vi "Do Core.vi"(8 "error in":errorcluster, 9 "Actor in":refnum<class "Actor.lvclass">, 11 "Reply Message":refnum<class "Get Pending IMatch Responses Reply Msg.lvclass">) -> (0 "error out":errorcluster, 1 "Actor out":refnum<class "Actor.lvclass">, 2 "Reply":variant)   [LabVIEW 2020, in "CANopen.lvlib" / "Response Matcher.lvlib" / "Get Pending IMatch Responses Reply Msg.lvclass"]
doc: "<p>(<strong>Filename</strong>: <span class=\"dnl\">Actor Framework.lvlib:Reply Msg.lvclass:Do Core.vi</span>)</p>\n<p>Defines what an actor does when it receives <strong>Reply Message</strong>. This method also defines the <strong>Reply</strong> that is returned to the actor that sent <strong>Reply Message</strong>.</p>\n<p>By default, this method does nothing, and <strong>Reply</strong> is the ancestor Message class. A child class must override this method to define behavior and specify a child of the Message class to return in the <strong>Reply</strong> output.</p>"
uses:
  Get Pending IMatch Responses Reply Msg.lvclass
  <vilib>/ActorFramework/Actor/Actor.lvclass
  Response Matcher/Response Matcher.lvclass
  C:/Program Files/National Instruments/LabVIEW 2026/vi.lib/ActorFramework/Actor/Actor.lvclass
  Response Matcher/Response Matcher.lvclass/Response Matcher.ctl
  IResponse/IMatch Response.lvclass
  Get Pending IMatch Responses Reply Msg.lvclass/Get Pending IMatch Responses Reply Msg.ctl
  9594798c-f666-4898-a9cb-e8de1dd19067.vi
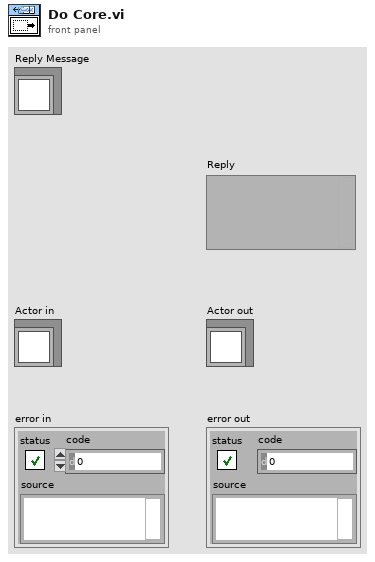
[diagram p1: front panel]
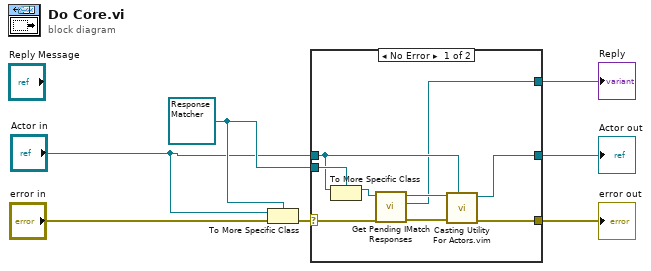
[diagram p0: block diagram]
diagram:
  w4 = refnum<class "Response Matcher.lvclass"> refnum ("CANopen.lvlib:Response Matcher.lvlib:Response Matcher")
  n1 = To More Specific Class(target class=w4, reference="Actor in", error in="error in") -> (error out=w7:errorcluster)  [unwired: 1 out]
  n2 = case shown="No Error" w7 {
    selector: w7 -> [w11 w18]
    tunnel: [w13 w18] -> w6
    tunnel: [w14 w17] -> w2
    tunnel: "Actor in" -> [w15 w17]
    tunnel: w4 -> [w16 _]
    tunnel: [w9 _] -> w1
    frame No Error {
      n3 = To More Specific Class(target class=w16, reference=w15) -> (specific class reference=w8:refnum<class "Response Matcher.lvclass">)  [unwired: 1 in, 1 out]
      n4 = call "Get Pending IMatch Responses.vi"("error in"=w11, "Response Matcher in"=w8) -> ("error out"=w12:errorcluster, "Pending IMatch Responses"=w9:refnum<data-value>, "Response Matcher out"=w10:refnum<class "Response Matcher.lvclass">)  [unwired: 7 in]
      n5 = call "Casting Utility For Actors.vim"("type"=w15, "error in (no error)"=w12, "Actor in"=w10) -> ("error out"=w13:errorcluster, "Actor out"=w14:refnum<class "Actor.lvclass">)  [unwired: 7 in]
    }
    frame Error {
      # "If type check fails, pass the original object out again."
    }
  }
  "error out" <- w6
  "Actor out" <- w2
  "Reply" <- w1
